vi "Measurement-LT.vi"(8 "Function (0: Cp-D)":u16(ring) items=["Cp-D", "Cp-Q", "Cp-G", "Cp-Rp", "Cs-D", "Cs-Q", "Cs-Rs", "Lp-D", "Lp-Q", "Lp-G", "Lp-Rp", "Lp-Rdc", "Ls-D", "Ls-Q", "Ls-Rs", "Ls-Rdc", "R-X", "Z-thd", "Z-thr", "G-B", "Y-thd", "Y-thr", "Vdc-Idc"], 9 "Cluster 2":T1={"客户仪器地址"="USB0::0x0471::0x2826::QF71600867::INSTR", "低温地址"="COM3", "BSFR"=refnum, "测试频率"={"数值"=0.0, "数值 2"=0.0, "数值 3"=0.0, "数值 4"=0.0}, "error in (no error)"={"status"=FALSE, "code"=0, "source"=""}, "结束温度"=100000.0, "开始温度"=100000.0}, 10 "Ctl Refnum 2":refnum<vi>, 11 "Ctl Refnum":refnum<vi>) -> (1 "Cluster":T2)   [LabVIEW 2017]
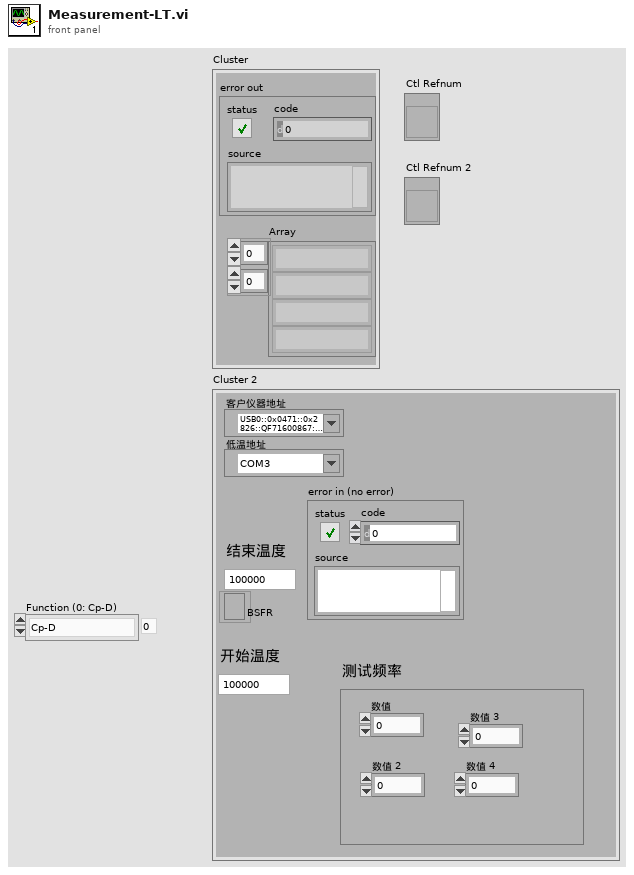
[diagram p1: front panel]
types:
  T1 = cluster{"客户仪器地址":refnum<visa-resource-name>, "低温地址":refnum<visa-resource-name>, "BSFR":refnum<file>, "测试频率":cluster{"数值":dbl, "数值 2":dbl, "数值 3":dbl, "数值 4":dbl}, "error in (no error)":errorcluster, "结束温度":dbl, "开始温度":dbl}
  T2 = cluster{"Array":string[][], "error out":errorcluster}
  T3 = cluster{"数值":dbl, "数值 2":dbl, "数值 3":dbl, "数值 4":dbl}
  T4 = cluster{"Array 2":string[][], "error out":errorcluster}
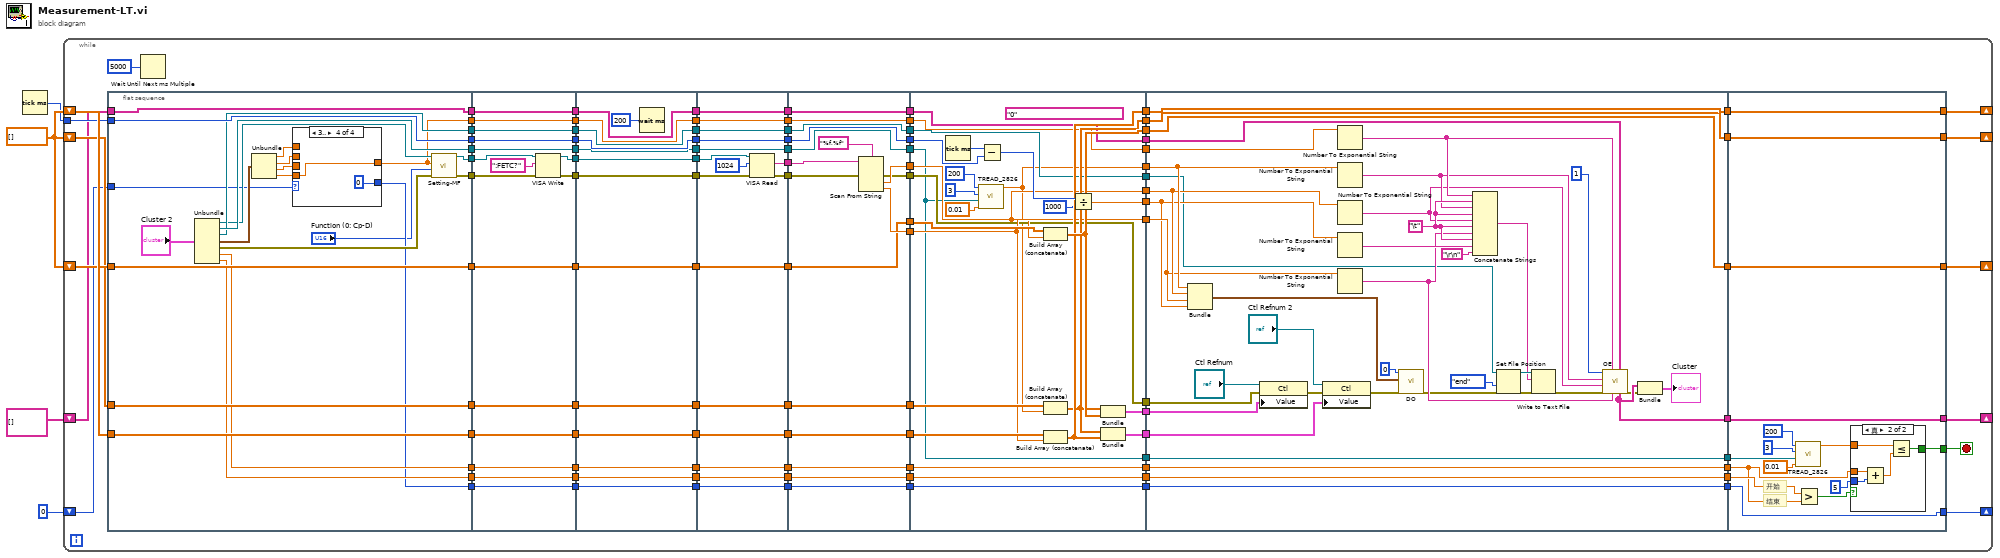
[diagram p0: block diagram]
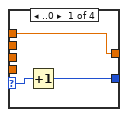
[diagram p2: hidden frame]
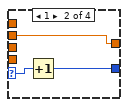
[diagram p3: hidden frame]
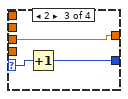
[diagram p4: hidden frame]
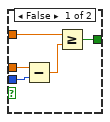
[diagram p5: hidden frame]
diagram:
  w4 = dbl[] []
  n1 = Tick Count (ms)() -> (millisecond timer value=w2:u32)
  n2 = while {
    tunnel: w2 -> [w65]
    shift-right: [w63] -> _
    shift-left: w4 -> [w68]
    shift-right: [w62] -> _
    shift-left: w4 -> [w66]
    shift-right: [w61] -> _
    shift-left: w4 -> [w67]
    shift-right: [w60] -> _
    shift-left: string[][] [] -> [w64]
    shift-right: [w18] -> _
    shift-left: 0 -> [w19]
    stop <- w49 stop-if-true
    n3 = flat-sequence {
      tunnel: w68 -> [w128]
      tunnel: w67 -> [w129]
      tunnel: w66 -> [w130]
      tunnel: w65 -> [w131]
      tunnel: [w131] -> w41
      tunnel: [w130] -> w39
      tunnel: [w129] -> w37
      tunnel: [w128] -> w35
      tunnel: [w127] -> w31
      tunnel: w64 -> [w127]
      tunnel: [w126] -> w29
      tunnel: [w125] -> w27
      tunnel: [w123] -> w25
      tunnel: [w122] -> w23
      tunnel: [w120] -> w21
      tunnel: [w118] -> w20
      tunnel: w19 -> [w116]
      tunnel: [w115] -> w11
      tunnel: [w110] -> w5
      tunnel: w41 -> [w158]
      tunnel: [w158] -> w40
      tunnel: w39 -> [w157]
      tunnel: [w157] -> w38
      tunnel: w37 -> [w156]
      tunnel: [w156] -> w36
      tunnel: w35 -> [w155]
      tunnel: [w155] -> w34
      tunnel: [w146] -> w33
      tunnel: [w147] -> w32
      tunnel: w31 -> [w154]
      tunnel: [w154] -> w30
      tunnel: w29 -> [w153]
      tunnel: [w153] -> w28
      tunnel: w27 -> [w152]
      tunnel: [w152] -> w26
      tunnel: w25 -> [w151]
      tunnel: [w151] -> w24
      tunnel: w23 -> [w150]
      tunnel: [w150] -> w22
      tunnel: w21 -> [w149]
      tunnel: w20 -> [w148]
      tunnel: [w144] -> w12
      tunnel: w11 -> [w144]
      tunnel: [w143] -> w6
      tunnel: w5 -> [w143]
      tunnel: [w172] -> w108
      tunnel: [w171] -> w107
      tunnel: [w170] -> w106
      tunnel: [w169] -> w105
      tunnel: w40 -> [w172]
      tunnel: w38 -> [w171]
      tunnel: w36 -> [w170]
      tunnel: w34 -> [w169]
      tunnel: [w167] -> w104
      tunnel: w33 -> [w167]
      tunnel: [w166] -> w103
      tunnel: w32 -> [w166]
      tunnel: [w165] -> w102
      tunnel: w30 -> [w165]
      tunnel: [w164] -> w101
      tunnel: w28 -> [w164]
      tunnel: [w163] -> w100
      tunnel: w26 -> [w163]
      tunnel: [w162] -> w56
      tunnel: w24 -> [w162]
      tunnel: [w161] -> w42
      tunnel: w22 -> [w161]
      tunnel: [w160] -> w13
      tunnel: w12 -> [w160]
      tunnel: [w159] -> w7
      tunnel: w6 -> [w159]
      tunnel: [w188] -> w99
      tunnel: [w187] -> w98
      tunnel: [w186] -> w97
      tunnel: [w185] -> w96
      tunnel: [w182] -> w95
      tunnel: [w183] -> w94
      tunnel: w108 -> [w188]
      tunnel: w107 -> [w187]
      tunnel: w106 -> [w186]
      tunnel: w105 -> [w185]
      tunnel: w104 -> [w181]
      tunnel: w103 -> [w180]
      tunnel: [w179] -> w93
      tunnel: w102 -> [w179]
      tunnel: [w178] -> w92
      tunnel: w101 -> [w178]
      tunnel: w100 -> [w177]
      tunnel: [w177] -> w91
      tunnel: [w176] -> w57
      tunnel: w56 -> [w176]
      tunnel: [w175] -> w43
      tunnel: w42 -> [w175]
      tunnel: [w174] -> w14
      tunnel: w13 -> [w174]
      tunnel: [w173] -> w8
      tunnel: w7 -> [w173]
      tunnel: [w202] -> w90
      tunnel: [w201] -> w89
      tunnel: [w200] -> w88
      tunnel: [w199] -> w87
      tunnel: [w204] -> w86
      tunnel: [w203] -> w85
      tunnel: [w198] -> w84
      tunnel: w99 -> [w202]
      tunnel: w98 -> [w201]
      tunnel: w97 -> [w200]
      tunnel: w96 -> [w199]
      tunnel: w95 -> [w197]
      tunnel: w94 -> [w196]
      tunnel: [w195] -> w83
      tunnel: w93 -> [w195]
      tunnel: [w194] -> w82
      tunnel: w92 -> [w194]
      tunnel: [w193] -> w81
      tunnel: w91 -> [w193]
      tunnel: [w192] -> w58
      tunnel: w57 -> [w192]
      tunnel: [w191] -> w44
      tunnel: w43 -> [w191]
      tunnel: [w190] -> w15
      tunnel: w14 -> [w190]
      tunnel: [w189] -> w9
      tunnel: w8 -> [w189]
      tunnel: w90 -> [w231]
      tunnel: w89 -> [w229]
      tunnel: w88 -> [w228]
      tunnel: w87 -> [w227]
      tunnel: [w226] -> w80
      tunnel: [w225] -> w79
      tunnel: [w224] -> w78
      tunnel: w86 -> [w221]
      tunnel: [w221] -> w77
      tunnel: w85 -> [w222]
      tunnel: [w222] -> w76
      tunnel: [w212] -> w75
      tunnel: [w209] -> w74
      tunnel: w84 -> [w218]
      tunnel: [w218] -> w73
      tunnel: w83 -> [w217]
      tunnel: [w217] -> w72
      tunnel: w82 -> [w211]
      tunnel: [w216] -> w71
      tunnel: w81 -> [w216]
      tunnel: [w215] -> w70
      tunnel: [w214] -> w69
      tunnel: w58 -> [w213]
      tunnel: [w213] -> w55
      tunnel: [w211] -> w48
      tunnel: [w208] -> w45
      tunnel: w44 -> [w208]
      tunnel: [w207] -> w16
      tunnel: w15 -> [w207]
      tunnel: [w206] -> w10
      tunnel: w9 -> [w206]
      tunnel: w80 -> [w265]
      tunnel: w79 -> [w264]
      tunnel: w78 -> [w263]
      tunnel: w77 -> [w261]
      tunnel: w76 -> [w260]
      tunnel: w75 -> [w262]
      tunnel: w74 -> [w259]
      tunnel: w73 -> [w247]
      tunnel: w72 -> [w257]
      tunnel: w71 -> [w252]
      tunnel: w70 -> [w245]
      tunnel: w69 -> [w244]
      tunnel: w55 -> [w240]
      tunnel: [w265] -> w54
      tunnel: [w264] -> w53
      tunnel: [w263] -> w52
      tunnel: [w251] -> w51
      tunnel: [w240] -> w50
      tunnel: w48 -> [w239]
      tunnel: [w239] -> w47
      tunnel: [w235] -> w46
      tunnel: w45 -> [w235]
      tunnel: [w234] -> w17
      tunnel: w16 -> [w234]
      tunnel: w10 -> [w233]
      tunnel: [w284] -> w60
      tunnel: [w285] -> w62
      tunnel: [w286] -> w63
      tunnel: [w287] -> w61
      tunnel: w54 -> [w287]
      tunnel: w53 -> [w286]
      tunnel: w52 -> [w285]
      tunnel: w51 -> [w284]
      tunnel: w50 -> [w277]
      tunnel: [w274] -> w49
      tunnel: w47 -> [w280]
      tunnel: w46 -> [w279]
      tunnel: [w273] -> w18
      tunnel: w17 -> [w273]
      frame #0 {
        n4 = Unbundle("Cluster 2") -> ("客户仪器地址"=w119:refnum<visa-resource-name>, "低温地址"=w126:refnum<visa-resource-name>, "BSFR"=w125:refnum<file>, "测试频率"=w117:T3, "error in (no error)"=w121:errorcluster, "结束温度"=w123:dbl, "开始温度"=w122:dbl)
        n5 = Unbundle(w117) -> ("数值"=w114:dbl, "数值 2"=w113:dbl, "数值 3"=w112:dbl, "数值 4"=w111:dbl)
        n6 = case shown="3.." w116 {
          selector: w116 -> [w134 w137 w140 _]
          tunnel: [w133 w136 w139 0] -> w115
          tunnel: [w132 w135 w138 w141] -> w110
          tunnel: w114 -> [w132 _ _ _]
          tunnel: w113 -> [_ w135 _ _]
          tunnel: w112 -> [_ _ w138 _]
          tunnel: w111 -> [_ _ _ w141]
          frame ..0 {
            n7 = Increment(x=w134) -> (x+1=w133:i32)
          }
          frame 1 {
            n8 = Increment(x=w137) -> (x+1=w136:i32)
          }
          frame 2 {
            n9 = Increment(x=w140) -> (x+1=w139:i32)
          }
          frame 3.. {
          }
        }
        n10 = call "Setting-MF.vi"("error in (no error)"=w121, "Function (0: Cp-D)"="Function (0: Cp-D)", "number"=w110, "VISA resource name"=w119) -> ("error out"=w120:errorcluster, "VISA resource name 2"=w118:refnum<visa-resource-name>)  [unwired: 6 in]
      }
      frame #1 {
        n11 = VISA Write(VISA resource name=w148, write buffer=":FETC?", error in (no error)=w149) -> (VISA resource name out=w146:refnum<visa-resource-name>, error out=w147:errorcluster)  [unwired: 1 out]
      }
      frame #2 {
        n12 = Wait (ms)(milliseconds to wait=u32 200 ("等待时间（毫秒）")) -> ()  [unwired: 1 out]
      }
      frame #3 {
        n13 = VISA Read(VISA resource name=w181, byte count=u32 1024 ("字节总数"), error in (no error)=w180) -> (read buffer=w182:string, error out=w183:errorcluster)  [unwired: 2 out]
      }
      frame #4 {
        n14 = Scan From String(format string="%f,%f" ("格式字符串"), input string=w197, error in=w196) -> (error out=w198:errorcluster, output 1=w204:dbl, output 2=w203:dbl)  [unwired: 3 in, 2 out]
      }
      frame #5 {
        (unwired) "0" ("Input Z format")
        n15 = Tick Count (ms)() -> (millisecond timer value=w232:u32)
        n16 = call "TREAD_2826.vi"("Unknown Param 2"=0.01, "VISA resource name"=w211, "Address No."=i8 3, "Unknown Param"=200) -> ("PV"=w212:dbl)  [unwired: 3 out]
        n17 = Subtract(x=w232, y=w231) -> (x-y=w230:u32)
        n18 = Build Array (concatenate)(w228, w221) -> (w226:dbl[])
        n19 = Build Array (concatenate)(w229, w212) -> (w224:dbl[])
        n20 = Build Array (concatenate)(w227, w222) -> (w225:dbl[])
        n21 = Divide(x=w230, y=u32 1000) -> (x/y=w209:dbl)
        n22 = Bundle(w224, w226) -> (w214:cluster{dbl[], dbl[]})  [unwired: 1 in]
        n23 = Bundle(w224, w225) -> (w215:cluster{dbl[], dbl[]})  [unwired: 1 in]
      }
      frame #6 {
        w267 = "\t"
        n24 = Bundle("PV"=w262, w261, w260, w259) -> (w250:cluster{"PV":dbl, dbl, dbl, dbl})  [unwired: 1 in]
        n25 = property class="Ctl"(reference="Ctl Refnum", error in=w247, "Value"=w244) -> (error out=w248:errorcluster)  [unwired: 1 out]
        n26 = property class="Ctl"(reference="Ctl Refnum 2", error in=w248, "Value"=w245) -> (error out=w246:errorcluster)  [unwired: 1 out]
        n27 = Number To Exponential String(number=w233) -> (E-format string=w256:string)  [unwired: 3 out]
        n28 = Number To Exponential String(number=w262) -> (E-format string=w255:string)  [unwired: 3 out]
        n29 = Number To Exponential String(number=w261) -> (E-format string=w254:string)  [unwired: 3 out]
        n30 = Number To Exponential String(number=w259) -> (E-format string=w266:string)  [unwired: 3 out]
        n31 = Number To Exponential String(number=w260) -> (E-format string=w253:string)  [unwired: 3 out]
        n32 = call "DO.vi"("error in (no error)"=w246, "数据输出"=w250, "功能编号"=0) -> ("error out"=w238:errorcluster)  [unwired: 8 in]
        n33 = Concatenate Strings(w256, w267, w255, w267, w254, w267, w253, w267, w266, "\r\n") -> (w270:string)
        n34 = Set File Position(refnum=w252, from (0:start)=enum16{"start", "end", "current"}."end" ("自（0:起始）"), error in=w238) -> (refnum out=w272:refnum<file>, error out=w269:errorcluster)  [unwired: 1 out]
        n35 = Write to Text File(file (use dialog)=w272, text=w270, error in=w269) -> (error out=w237:errorcluster)  [unwired: 3 out]
        n36 = call "OE.vi"("Array"=w257, "String 4"=w253, "String"=w256, "error in (no error)"=w237, "String 3"=w254, "String 2"=w255, "Numeric"=1) -> ("error out"=w236:errorcluster, "Array 2"=w251:string[][])  [unwired: 2 in, 1 out]
        n37 = Bundle("Array 2"=w251, "error out"=w236) -> (→"Cluster":T4)  [unwired: 1 in]
      }
      frame #7 {
        # "结束"
        # "开始"
        n38 = call "TREAD_2826.vi"("Unknown Param 2"=0.01, "VISA resource name"=w280, "Address No."=i8 3, "Unknown Param"=200) -> ("PV"=w275:dbl)  [unwired: 3 out]
        n39 = Greater?(x=w279, y=w277) -> (0:w278:bool)
        n40 = case shown="真" w278 {
          tunnel: w277 -> [w292 w297]
          tunnel: 5 -> [w291 w296]
          tunnel: w275 -> [w290 w295]
          tunnel: [w288 w293] -> w274
          frame False {
            n41 = Subtract(x=w292, y=w291) -> (x-y=w289:dbl)
            n42 = Greater Or Equal?(x=w290, y=w289) -> (x >= y?=w288:bool)
          }
          frame True {
            n43 = Add(x=w297, y=w296) -> (x+y=w294:dbl)
            n44 = Less Or Equal?(x=w295, y=w294) -> (x <= y?=w293:bool)
          }
        }
      }
    }
    n45 = Wait Until Next ms Multiple(millisecond multiple=u32 5000 ("毫秒倍数")) -> ()  [unwired: 1 out]
  }
